vi "SYST_ERR.vi"(0 "VISA IN":refnum<visa-resource-name>, 5 "error in":errorcluster) -> (14 "VISA Out":refnum<visa-resource-name>, 16 "Data":string, 19 "error out":errorcluster)   [LabVIEW 2018, in "PNA-X.lvlib"]
doc: "SYSTem:ERRor? \n(Read-only) Returns the next error in the error queue. Each time the analyzer detects an error, it places \na message in the error queue. When the SYSTEM:ERROR? query is sent, one message is moved from \nthe error queue to the output queue so it can be read by the controller. Error messages are delivered to \nthe output queue in the order they were received. The error queue is cleared when any of the following \nconditions occur: \nWhen the analyzer is switched ON. \nWhen the *CLS command is sent to the analyzer. \nWhen all of the errors are read. \nIf the error queue overflows, the last error is replaced with a \"Queue Overflow\" error. The \noldest errors remain in the queue and the most recent error is discarded. \nExamples SYST:ERR? \nsystem:error? \nDefault Not Applicable"
uses:
  PNA-X.lvlib
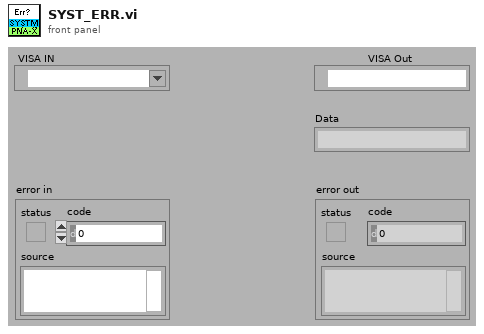
[diagram p1: front panel]
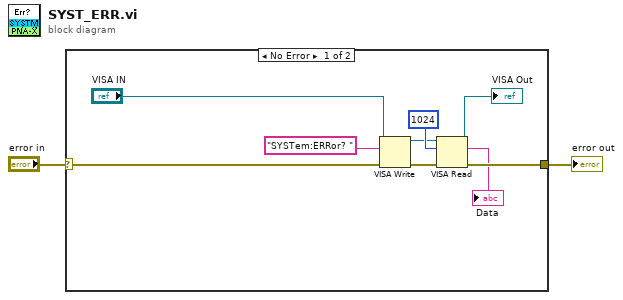
[diagram p0: block diagram]
diagram:
  n1 = case shown="No Error" "error in" {
    selector: "error in" -> [w4 w12]
    tunnel: [w7 w12] -> w1
    frame No Error {
      n2 = VISA Write(VISA resource name="VISA IN", write buffer="SYSTem:ERRor? " ("Cmdline"), error in (no error)=w4) -> (VISA resource name out=w8:refnum<visa-resource-name>, error out=w10:errorcluster)  [unwired: 1 out]
      n3 = VISA Read(VISA resource name=w8, byte count=1024, error in (no error)=w10) -> (VISA resource name out=→"VISA Out":refnum<visa-resource-name>, read buffer=→"Data":string, error out=w7:errorcluster)  [unwired: 1 out]
    }
    frame Error {
    }
  }
  "error out" <- w1
